vi "logAppliedSettingsMatchStart.vi"(8 "error in (no error)":errorcluster, 10 "EventAppliedSettingsMatchStart":T1, 11 "M1M3SAL in":refnum<class "M1M3SAL.lvclass">) -> (0 "error out":errorcluster, 3 "M1M3SAL out":refnum<class "M1M3SAL.lvclass">)   [LabVIEW 2016, in "M1M3SupportCommunicator.lvlib" / "M1M3SAL.lvclass"]
uses:
  M1M3SAL.lvclass
  DataTypes/Topics/EventAppliedSettingsMatchStart.ctl
  DataTypes/Topics/Parts/Timestamp.ctl
  DataTypes/MessageHeader.ctl
  DataTypes/MessageTypes.ctl
  DataTypes/MessageTopics.ctl
  M1M3SAL.lvclass/M1M3SAL.ctl
  writeU8.vi
  M1M3SupportCommunicator.lvlib
  DataTypes/Topics/M1M3SupportTopics.lvlib
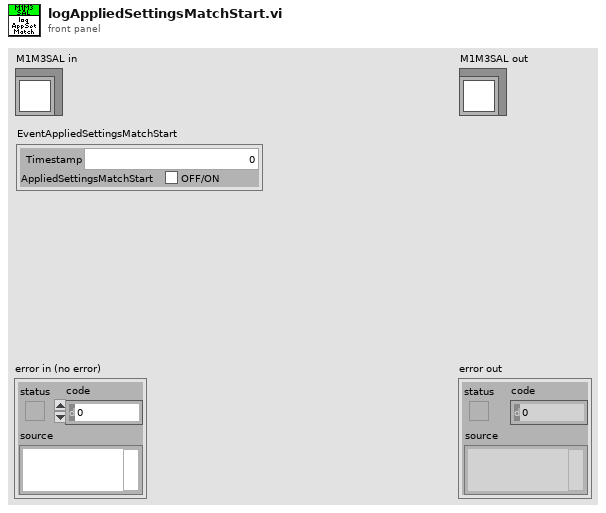
[diagram p1: front panel]
types:
  T1 = typedef "M1M3SupportTopics.lvlib/EventAppliedSettingsMatchStart.ctl" = cluster{"Timestamp":T2, "AppliedSettingsMatchStart":bool}
  T2 = typedef "M1M3SupportTopics.lvlib/Timestamp.ctl" = dbl
  T3 = typedef "M1M3SupportCommunicator.lvlib/MessageHeader.ctl" = cluster{"Type":T4, "Topic":T5, "Size":i32}
  T4 = typedef "M1M3SupportCommunicator.lvlib/MessageTypes.ctl" = enum8{"None", "PutSample", "GetNextSample", "LogEvent", "GetEvent", "IssueCommand", "CommandId", "WaitForCompletion", "AcceptCommand", "AckCommand"}
  T5 = typedef "M1M3SupportCommunicator.lvlib/MessageTopics.ctl" = enum8{"None", "ForceActuatorData", "MirrorForceData", "HardpointData", "AirData", "DynamicData", "FPGAData", "IMSData", "ForceActuatorStatus", "ElevationData", "HardpointStatus", "HardpointActuatorChase", "AirStatus", "ForceActuatorSafetyChecks", "ForceActuatorTest", "ActuatorBroadcastCounter", "StatusChecks", "CellChecks", "HardpointActuatorBreakaway", "RaiseMirrorComplete", "ILCCommunication", "ElevationAngleChecks", "DetailedState", "ServoLoops", "ForceActuatorInfo", "LowerMirrorComplete", "HardpointActuatorInfo", "SettingsApplied", "ErrorCode", "StartupChecks", "SummaryState", "SettingVersions", "ActuatorTestStatus", "AppliedSettingsMatchStart", "Enable", "EnterMaintenance", "Standby", "AbortLowerM1M3", "ApplyAberrationByForces", "ApplyAOSCorrectionByBendingModes", "ClearAOSCorrection", "Start", "RaiseM1M3", "TestForceActuator", "LowerM1M3", "ApplyAOSCorrectionByForces", "Disable", "ApplyAberationByBendingMode", "TestHardpoint", "ManipulateM1M3", "ClearAberration", "Exit", "TestAir", "AbortRaiseM1M3", "MoveHardpointActuators", "ExitMaintenance", "Shutdown"}
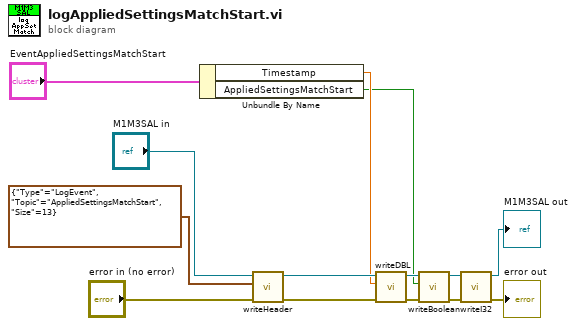
[diagram p0: block diagram]
diagram:
  n1 = Unbundle By Name("EventAppliedSettingsMatchStart") -> ("Timestamp"=w2:T2, "AppliedSettingsMatchStart"=w1:bool)
  n2 = call "writeHeader.vi"("error in (no error)"="error in (no error)", "MessageHeader"=T3 {"Type"=enum."LogEvent", "Topic"=enum."AppliedSettingsMatchStart", "Size"=13}, "M1M3SAL in"="M1M3SAL in") -> ("error out"=w10:errorcluster, "M1M3SAL out"=w6:refnum<class "M1M3SAL.lvclass">)  [unwired: 7 in]
  n3 = call "writeDBL.vi"("error in (no error)"=w10, "Input"=w2, "M1M3SAL in"=w6) -> ("error out"=w9:errorcluster, "M1M3SAL out"=w5:refnum<class "M1M3SAL.lvclass">)  [unwired: 7 in]
  n4 = call "writeBoolean.vi"("error in (no error)"=w9, "Input"=w1, "M1M3SAL in"=w5) -> ("error out"=w8:errorcluster, "M1M3SAL out"=w4:refnum<class "M1M3SAL.lvclass">)  [unwired: 7 in]
  n5 = call "writeI32.vi"("error in (no error)"=w8, "M1M3SAL in"=w4) -> ("error out"=→"error out":errorcluster, "M1M3SAL out"=→"M1M3SAL out":refnum<class "M1M3SAL.lvclass">)  [unwired: 8 in]
